vi "PH_Beckhoff_StepMot.set Settings.vi"(0 "VI in":refnum<vi>, 1 "AMS Net ID in":T1, 2 "Axis":i32, 3 "ADS Error in":i32, 4 "Step Motor Configuration":T2, 5 "error in (no error)":errorcluster) -> (14 "VI out":refnum<vi>, 15 "AMS Net ID out":T1, 16 "Settings changed?":bool, 17 "ADS Error out":i32, 18 "ok?":bool, 19 "error out":errorcluster)   [LabVIEW 2014, in "PH_Beckhoff_StepMot.lvlib"]
uses:
  PH_Beckhoff_StepMot.lvlib
  instr.lib/Beckhoff/Specials/Step Motor Klemmen/Beckhoff.Step Motor - Motor Configuration.ctl
  instr.lib/Beckhoff/Read and Write Register/Step Motor Klemmen/Beckhoff.Step Motor - Feature Register 1.ctl
  instr.lib/Beckhoff/Read and Write Register/Step Motor Klemmen/Beckhoff.Step Motor - Feature Register 2.ctl
  instr.lib/Beckhoff/Helpers/Beckhoff Access.ctl
  PH_Beckhoff_StepMot.Axis Cluster.ctl
  instr.lib/Beckhoff/Beckhoff - Driver np.lvlib
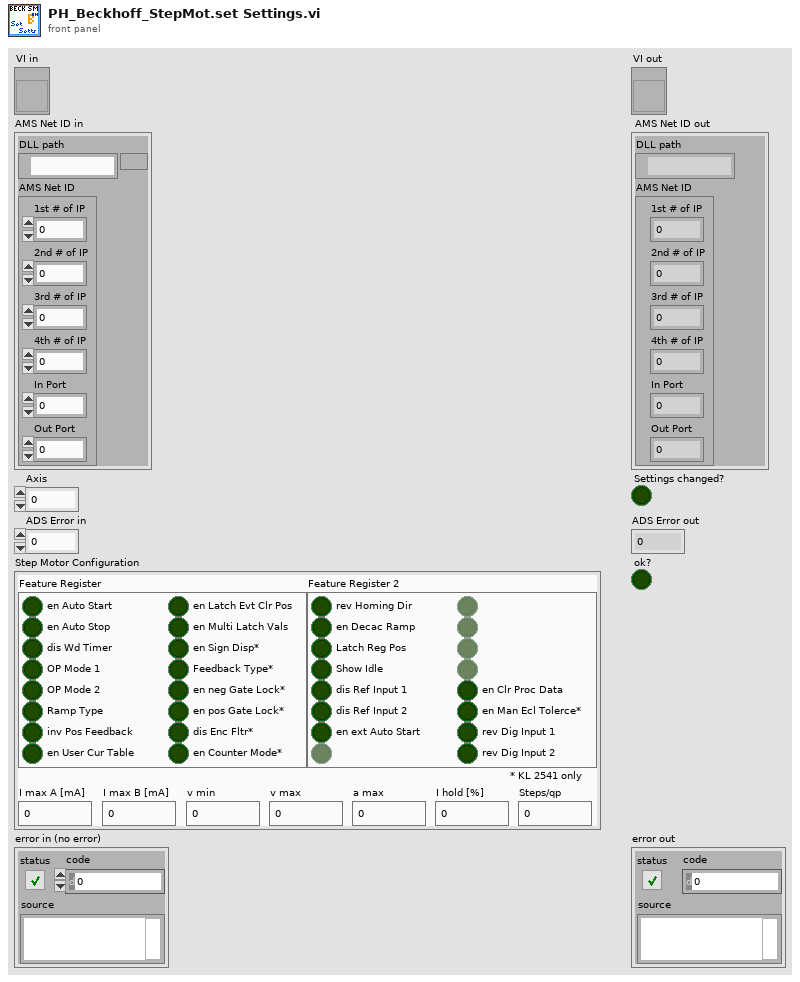
[diagram p1: front panel]
types:
  T1 = typedef "Beckhoff - Driver np.lvlib/Beckhoff Access.ctl" = cluster{"DLL path":path, "AMS Net ID":cluster{"1st # of IP":u8, "2nd # of IP":u8, "3rd # of IP":u8, "4th # of IP":u8, "In Port":u8, "Out Port":u8}}
  T2 = typedef "Beckhoff - Driver np.lvlib/Beckhoff.Step Motor - Motor Configuration.ctl" = cluster{"Feature Register":T3, "I max A [mA]":dbl, "I max B [mA]":dbl, "v min":u32, "v max":u32, "a max":u32, "I hold [%]":u32, "Steps/qp":u32, "Feature Register 2":T4}
  T3 = typedef "Beckhoff - Driver np.lvlib/Beckhoff.Step Motor - Feature Register 1.ctl" = cluster{"en Auto Start":bool, "en Auto Stop":bool, "dis Wd Timer":bool, "OP Mode 1":bool, "OP Mode 2":bool, "Ramp Type":bool, "inv Pos Feedback":bool, "en User Cur Table":bool, "en Latch Evt Clr Pos":bool, "en Multi Latch Vals":bool, "en Sign Disp*":bool, "Feedback Type*":bool, "en neg Gate Lock*":bool, "en pos Gate Lock*":bool, "dis Enc Fltr*":bool, "en Counter Mode*":bool}
  T4 = typedef "Beckhoff - Driver np.lvlib/Beckhoff.Step Motor - Feature Register 2.ctl" = cluster{"rev Homing Dir":bool, "en Decac Ramp":bool, "Latch Reg Pos":bool, "Show Idle":bool, "dis Ref Input 1":bool, "dis Ref Input 2":bool, "en ext Auto Start":bool, "N/A":bool, "N/A":bool, "N/A":bool, "N/A":bool, "N/A":bool, "en Clr Proc Data":bool, "en Man Ecl Tolerce*":bool, "rev Dig Input 1":bool, "rev Dig Input 2":bool}
  T5 = typedef "PH_Beckhoff_StepMot.lvlib/PH_Beckhoff_StepMot.Axis Cluster.ctl" = cluster{"Step Motor Configuration":T2, "To set?":bool, "Endswitch inverted?":bool}
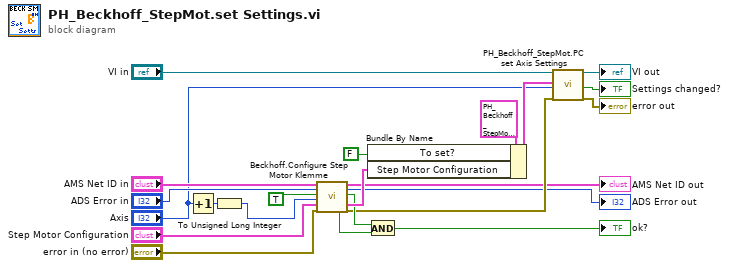
[diagram p0: block diagram]
diagram:
  n1 = Increment(x="Axis") -> (x+1=w3:i32)
  n2 = To Unsigned Long Integer(number=w3) -> (unsigned 32bit integer=w2:u32)
  n3 = call "Beckhoff.Configure Step Motor Klemme.vi"("AMS Net ID in"="AMS Net ID in", "ADS Error in"="ADS Error in", "Configure?"=TRUE ("Boolean in"), "Klemme"=w2, "Default Configuration"="Step Motor Configuration", "error in (no error)"="error in (no error)") -> ("Successfully configured?"=w13:bool, "AMS Net ID out"=→"AMS Net ID out":T1, "ADS Error out"=→"ADS Error out":i32, "Operation successful?"=w14:bool, "Current Step Motor Configuration"=w19:T2, "error out"=w9:errorcluster)  [unwired: 7 in, 1 out]
  n4 = Bundle By Name(cluster=T5 {"Step Motor Configuration"={"Feature Register"={"en Auto Start"=FALSE, "en Auto Stop"=FALSE, "dis Wd Timer"=FALSE, "OP Mode 1"=FALSE, "OP Mode 2"=FALSE, "Ramp Type"=FALSE, "inv Pos Feedback"=FALSE, "en User Cur Table"=FALSE, "en Latch Evt Clr Pos"=FALSE, "en Multi Latch Vals"=FALSE, "en Sign Disp*"=FALSE, "Feedback Type*"=FALSE, "en neg Gate Lock*"=FALSE, "en pos Gate Lock*"=FALSE, "dis Enc Fltr*"=FALSE, "en Counter Mode*"=FALSE}, "I max A [mA]"=0.0, "I max B [mA]"=0.0, "v min"=0, "v max"=0, "a max"=0, "I hold [%]"=0, "Steps/qp"=0, "Feature Register 2"={"rev Homing Dir"=FALSE, "en Decac Ramp"=FALSE, "Latch Reg Pos"=FALSE, "Show Idle"=FALSE, "dis Ref Input 1"=FALSE, "dis Ref Input 2"=FALSE, "en ext Auto Start"=FALSE, "N/A"=FALSE, "N/A"=FALSE, "N/A"=FALSE, "N/A"=FALSE, "N/A"=FALSE, "en Clr Proc Data"=FALSE, "en Man Ecl Tolerce*"=FALSE, "rev Dig Input 1"=FALSE, "rev Dig Input 2"=FALSE}}, "To set?"=FALSE, "Endswitch inverted?"=FALSE} ("Axis Settings"), "To set?"=FALSE, "Step Motor Configuration"=w19) -> (w20:T5)
  n5 = And(x=w14, y=w13) -> (x .and. y?=→"ok?":bool)
  n6 = call "PH_Beckhoff_StepMot.PC set Axis Settings.vi"("VI in"="VI in", "Axis Settings"=w20, "Axis"="Axis", "error in (no error)"=w9) -> ("VI out"=→"VI out":refnum<vi>, "Settings changed?"=→"Settings changed?":bool, "error out"=→"error out":errorcluster)  [unwired: 13 in]
